vi "SeaCOM-7203.vi"() -> ()   [LabVIEW 2020]
uses:
  <vilib>/Utility/miscctls.llb/LVPointTypeDef.ctl
  LabVIEW 2020 Toolkits/toolkits_lv2020_32bit/Synchronization.llb/SynchRefs_SetGet.ctl
  LabVIEW 2020 Toolkits/VI Server Toolkit/VI Server Libraries/VI Server_GetControl.llb/VI Server_STR_Get.vi
  LabVIEW 2020 Toolkits/VI Server Toolkit/VI Server Libraries/VI Server_Set Controls.llb/Set STR Control.vi
  LabVIEW 2020 Toolkits/VI Server Toolkit/VI Server Libraries/VI Server_GetControl.llb/VI Server_1D_Array_DBL_Get.vi
  LabVIEW 2020 Toolkits/VI Server Toolkit/VI Server Libraries/VI Server_GetControl.llb/VI Server_I32_Get.vi
  LabVIEW 2020 Toolkits/VI Server Toolkit/VI Server Libraries/VI Server_SetControl.llb/VI Server_DBL_Set.vi
  LabVIEW 2020 Toolkits/VI Server Toolkit/VI Server Libraries/VI Server_SetControl.llb/VI Server_U8_Set.vi
  LabVIEW 2020 Toolkits/VI Server Toolkit/VI Server Libraries/VI Server_SetControlValue_ArrayInputs.llb/VI Server_Set U8s From ArrayInputs.vi
  LabVIEW 2020 Toolkits/VI Server Toolkit/VI Server Libraries/VI Server_SetControl.llb/VI Server_1D_STR_Set.vi
  LabVIEW 2020 Toolkits/VI Server Toolkit/VI Server Libraries/VI Server_GetControl.llb/VI Server_1D_Array_STR_Get.vi
  LabVIEW 2020 Toolkits/VI Server Toolkit/VI Server Toolkit LV2013.lvlib
panel:
  in  "Manual.Open":bool caption="IDD.Open"
  in  "IDD.Open":bool
  in  "Help":bool
  in  "FP.Hide":bool caption="FrontPanel.Hide"
  out "System.Message":string caption="System Message"
  in  "EXIT":bool
  in  "Tab.Main":T1(tab)
  out "Ch2.ReceivedDataArray.IndexedValue":dbl caption="Value" format="%0.0f"
  in  "Ch2.ReceivedDataArray.Index":i32 caption="Index" max=6
  in  "Ch2.ReceivedDataArray.Precision":u8 caption="Precision" max=6
  out "Ch2.ReceivedDataArray":dbl[](array[numeric]) caption="Received Data Array"
  out "Ch2.Responce.String":string
  out "Ch2.Responce.Payload.Num4":dbl caption="Payload Numeric 4"
  out "Ch2.Responce.Payload.Num3":dbl caption="Payload Numeric 3"
  out "Ch2.Responce.Payload.Num2":dbl caption="Payload Numeric 2"
  out "Ch2.Responce.Payload.Num1":dbl caption="Payload Numeric 1"
  out "Ch1.ReceivedDataArray.IndexedValue":dbl caption="Value" format="%0.0f"
  in  "Ch1.ReceivedDataArray.Index":i32 caption="Index" max=6
  in  "Ch1.ReceivedDataArray.Precision":u8 caption="Precision" max=6
  out "Ch1.ReceivedDataArray":dbl[](array[numeric]) caption="Received Data Array"
  out "Ch1.Responce.String":string
  out "Ch2.Responce.Message.Checksum":string caption="Checksum"
  out "Ch2.Responce.Message.Load":string caption="PayloadLoad"
  out "Ch2.Responce.Message.Length":string caption="Length"
  out "Ch2.Responce.Message.ID":string caption="Message ID"
  out "Ch2.Responce.Message.Payload":u8[](array[numeric]) caption="Message Payload" format="%02x"
  out "Ch1.Responce.Payload.Num4":dbl caption="Payload Numeric 4"
  out "Ch1.Responce.Payload.Num3":dbl caption="Payload Numeric 3"
  out "Ch1.Responce.Payload.Num2":dbl caption="Payload Numeric 2"
  out "Ch1.Responce.Payload.Num1":dbl caption="Payload Numeric 1"
  out "Ch1.Responce.Message.Checksum":string caption="Checksum"
  out "Ch1.Responce.Message.Load":string caption="PayloadLoad"
  out "Ch1.Responce.Message.Length":string caption="Length"
  out "Ch1.Responce.Message.ID":string caption="Message ID"
  out "Ch1.Responce.Message.Payload":u8[](array[numeric]) caption="Message Payload" format="%02x"
  out "StringMode.Received Data":string
  in  "Argument.Update":bool
  in  "Argument.Precision":u8 caption="Precision" max=6
  in  "Argument.Value":dbl caption="Value"
  in  "Argument.Number":i32=1 caption="Number" min=1 max=100
  in  "Message.PrototypeString":string caption="Message Prototype String"
  in  "Protocol.MessageType":u16(ring) caption="Message Type" items=["Binary", "String"]
  out "Responce.Payload.Num4":dbl caption="Payload Numeric 4"
  out "Responce.Payload.Num3":dbl caption="Payload Numeric 3"
  out "Responce.Payload.Num2":dbl caption="Payload Numeric 2"
  out "Responce.Payload.Num1":dbl caption="Payload Numeric 1"
  out "Responce.Message.Checksum":string caption="Checksum"
  out "Responce.Message.Load":string caption="PayloadLoad"
  out "Responce.Message.Length":string caption="Length"
  out "Responce.Message.ID":string caption="Message ID"
  out "Responce.Message.Payload":u8[](array[numeric]) caption="Message Payload" format="%02x"
  in  "Protocol.New":string caption="New Protocol"
  in  "Message.ItemName.Delete":bool
  in  "Protocol.ADD":bool
  in  "Protocol":u16(ring) items=["Motion Controller"]
  in  "Protocol.Delete":bool
  in  "Message.Checksum.Skip":bool
  in  "Message.Checksum":u8 caption="Checksum" format="%02x"
  in  "Message.Payload.Length":u8 caption="Payload Length" format="%02x"
  in  "Message.ID":u8 caption="ID" format="%02x"
  in  "Message.ItemName":string caption="Item Name"
  in  "Message.String.Send":bool
  in  "Message.String.Regenerate":bool
  in  "Configuration.Message.Reload":bool
  in  "Configuration.Message.SAVE":bool
  in  "Message.String":string caption="Message String"
  in  "Message.ItemName.ADD":bool caption="Message.ItemName.Update"
  in  "Message":u16(ring) caption="Messages" items=["Move Absolute Position", "Move Relative Position"]
  in  "Message.Payload":u8[](array[numeric]) caption="Message Payload" format="%02x"
  in  "Channel":u16(ring) items=["Ch1", "Ch2"]
  in  "Message.String.Send.DUP":bool caption="Message.String.Send"
  in  "Ch1.Data.Autostroll":bool
  in  "Ch1.DataReceived.Clear":bool
  in  "Ch1.DataSent.Clear":bool
  out "Ch1.DataSent":string[](array[string]) caption="Data Sent"
  out "Ch1.DataReceived":string[](array[string]) caption="Data Received"
  in  "Message.String.Send.DUP1":bool caption="Message.String.Send"
  out "Ch2.DataSent":string[](array[string]) caption="Data Sent"
  out "Ch2.DataReceived":string[](array[string]) caption="Data Received"
  in  "Ch2.DataSent.Clear":bool
  in  "Ch2.Data.Autostroll":bool
  in  "Ch2.DataReceived.Clear":bool
  in  "Conversion.U32.Byte3":u8 caption="U8: Byte 3"
  in  "Conversion.U32.Byte2":u8 caption="U8: Byte 2"
  in  "Conversion.U2.Byte1":u8 caption="U8: Byte 1"
  in  "Conversion.U32.Byte0":u8 caption="U8: Byte 0"
  in  "Conversion.U32":u16 caption="U32"
  in  "Conversion.U8.LowerByte":u8 caption="U8: Lower Byte" format="%02x"
  in  "Conversion.U8.UpperByte":u8 caption="U8: Upper Byte" format="%02x"
  in  "Conversion.U16":u16 caption="U16"
  in  "Ch2.Stop.Bits":u16(ring)=1 caption="Stop Bits" items=["1.0"=10, "1.5"=15, "2.0"=20]
  in  "Ch2.Baud.Rate":u32=115200 caption="Baud Rate"
  in  "Ch2.Data.Bits":u16=8 caption="Data Bits" min=5 max=8 step=1
  in  "Ch2.Flow.Control":u16(ring) caption="Flow Control" items=["None", "XON/XOFF", "RTS/CTS", "XON/XOFF & RTS/CTS", "DTR/DSR", "XON/XOFF & DTR/DSR"]
  in  "Ch2.Parity":u16(ring) caption="Parity" items=["None", "Odd", "Even", "Mark", "Space"]
  in  "Ch2.VISA.Resource.Name":refnum<visa-resource-name>="COM4" caption="VISA Resource Name"
  in  "Ch1.Baud.Rate":u32=115200 caption="Baud Rate"
  in  "Ch1.Data.Bits":u16=8 caption="Data Bits" min=5 max=8 step=1
  in  "Ch1.Stop.Bits":u16(ring)=1 caption="Stop Bits" items=["1.0"=10, "1.5"=15, "2.0"=20]
  in  "Ch1.Flow.Control":u16(ring) caption="Flow Control" items=["None", "XON/XOFF", "RTS/CTS", "XON/XOFF & RTS/CTS", "DTR/DSR", "XON/XOFF & DTR/DSR"]
  in  "Ch1.Parity":u16(ring) caption="Parity" items=["None", "Odd", "Even", "Mark", "Space"]
  in  "Ch1.VISA.Resource.Name":refnum<visa-resource-name>="COM3" caption="VISA Resource Name"
  in  "Setup.AdobeAcrobat.Path":path=path "C:/Program Files (x86)/Adobe/Acrobat Reader DC/Reader/AcroRd32.exe" caption="Acrobat Reader Path"
  in  "VI.WindowsTitle":string caption="Windows Title"
  in  "UDP.Test.String2.Send":bool
  in  "UDP.Test.String2":string caption="UDP: Test String 2"
  in  "UDP.Port.BC":u16=58433 caption="UDP: Port.BC"
  in  "UDP.Port.RT":u16=58432 caption="UDP: Port.RT"
  in  "UDP.LocalPort.Write":u16=58434 caption="UDP: Local Port.Write"
  in  "UDP.IP.Address":string="234.5.6.7" caption="UDP: IP Address"
  in  "UDP.Test.String1.Send":bool
  in  "UDP.Test.String1":string caption="UDP: Test String 1"
  in  "UDP.Responce.String.Monitor":bool
  out "UDP.ExecEng.Message.String":string caption="UDP: Execution Engine Message String"
  out "error out":errorcluster
  in  "error in":errorcluster
  # "Channel 1 Received Data"
  # "Channel 2 Received Data"
  # "Received Data"
  # "Channel 2"
  # "Channel 1"
  # "Multicast IP addresses must be in the 224.0.0.0 to 239.255.255.255 range."
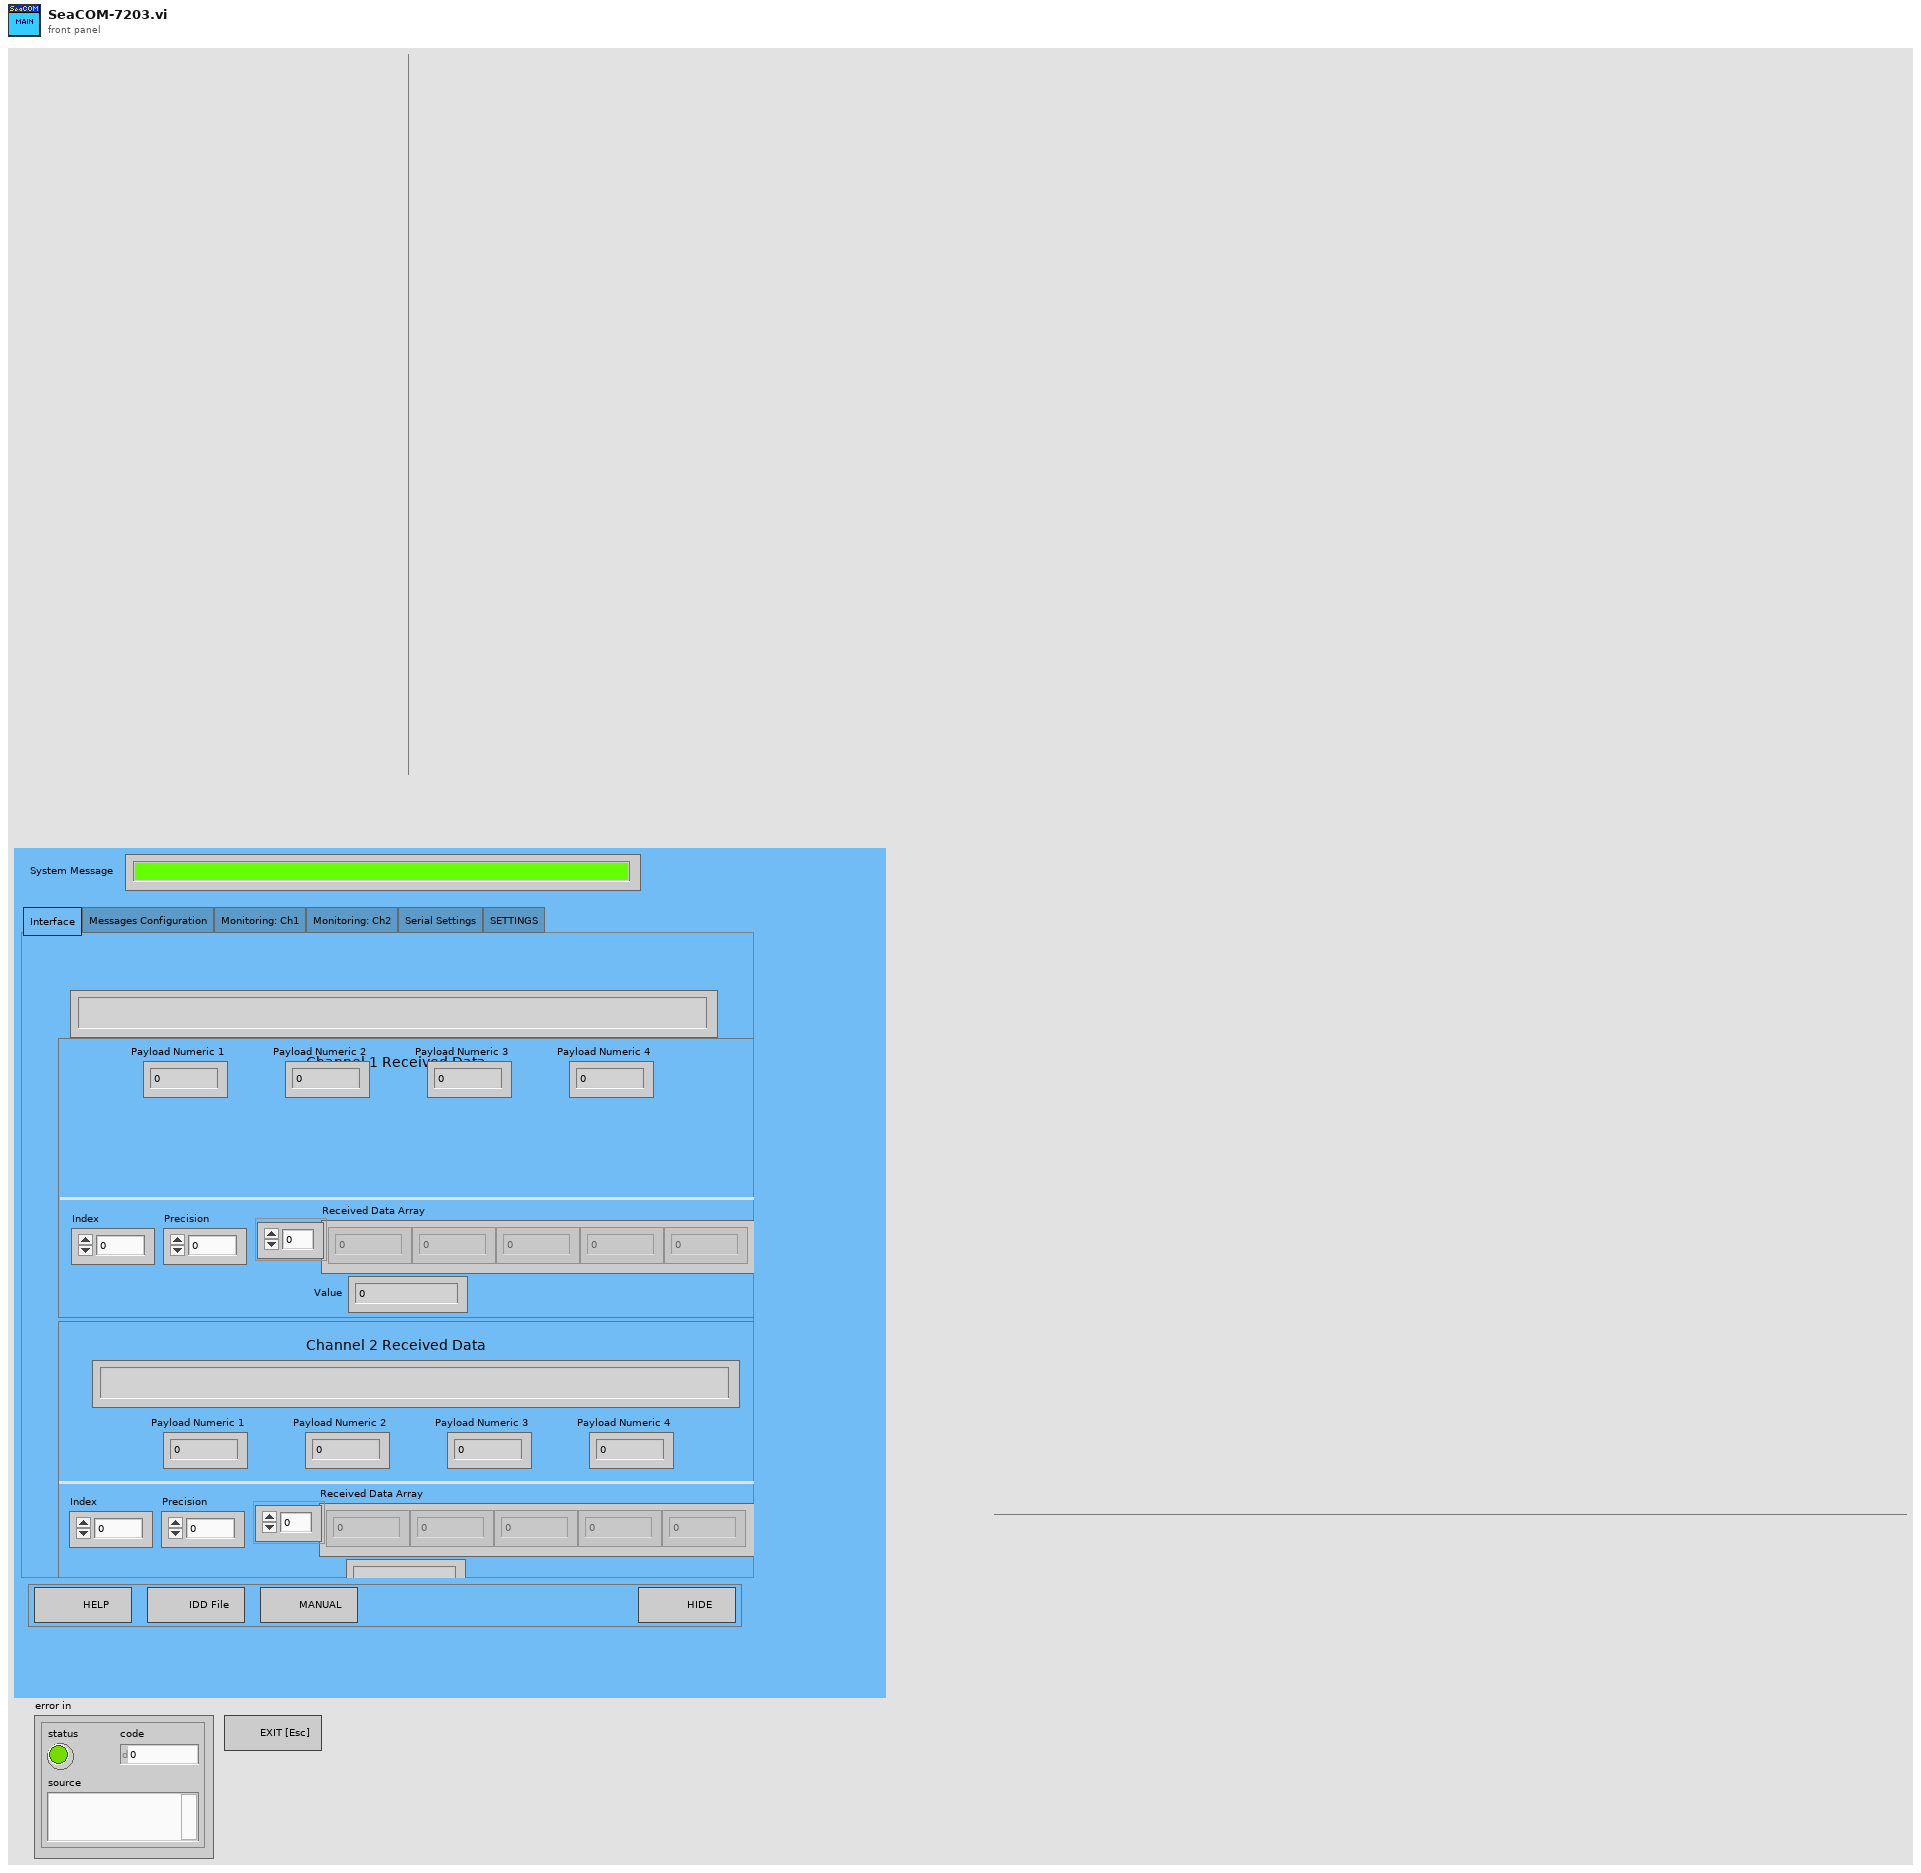
[diagram p1: front panel]
types:
  T1 = enum32{"Interface", "Messages Configuration", "Monitoring: Ch1", "Monitoring: Ch2", "Serial Settings", "SETTINGS"}
  T2 = typedef "LVPointTypeDef.ctl" = cluster{"Horizontal":i16, "Vertical":i16}
  T3 = typedef "VI Server_RefsCluster.ctl" = cluster{"Labels":string[], "Refs":refnum<vi>[], "VI Ref":refnum<vi>}
  T4 = typedef "SynchRefs_SetGet.ctl" = enum16{"Set", "Get"}
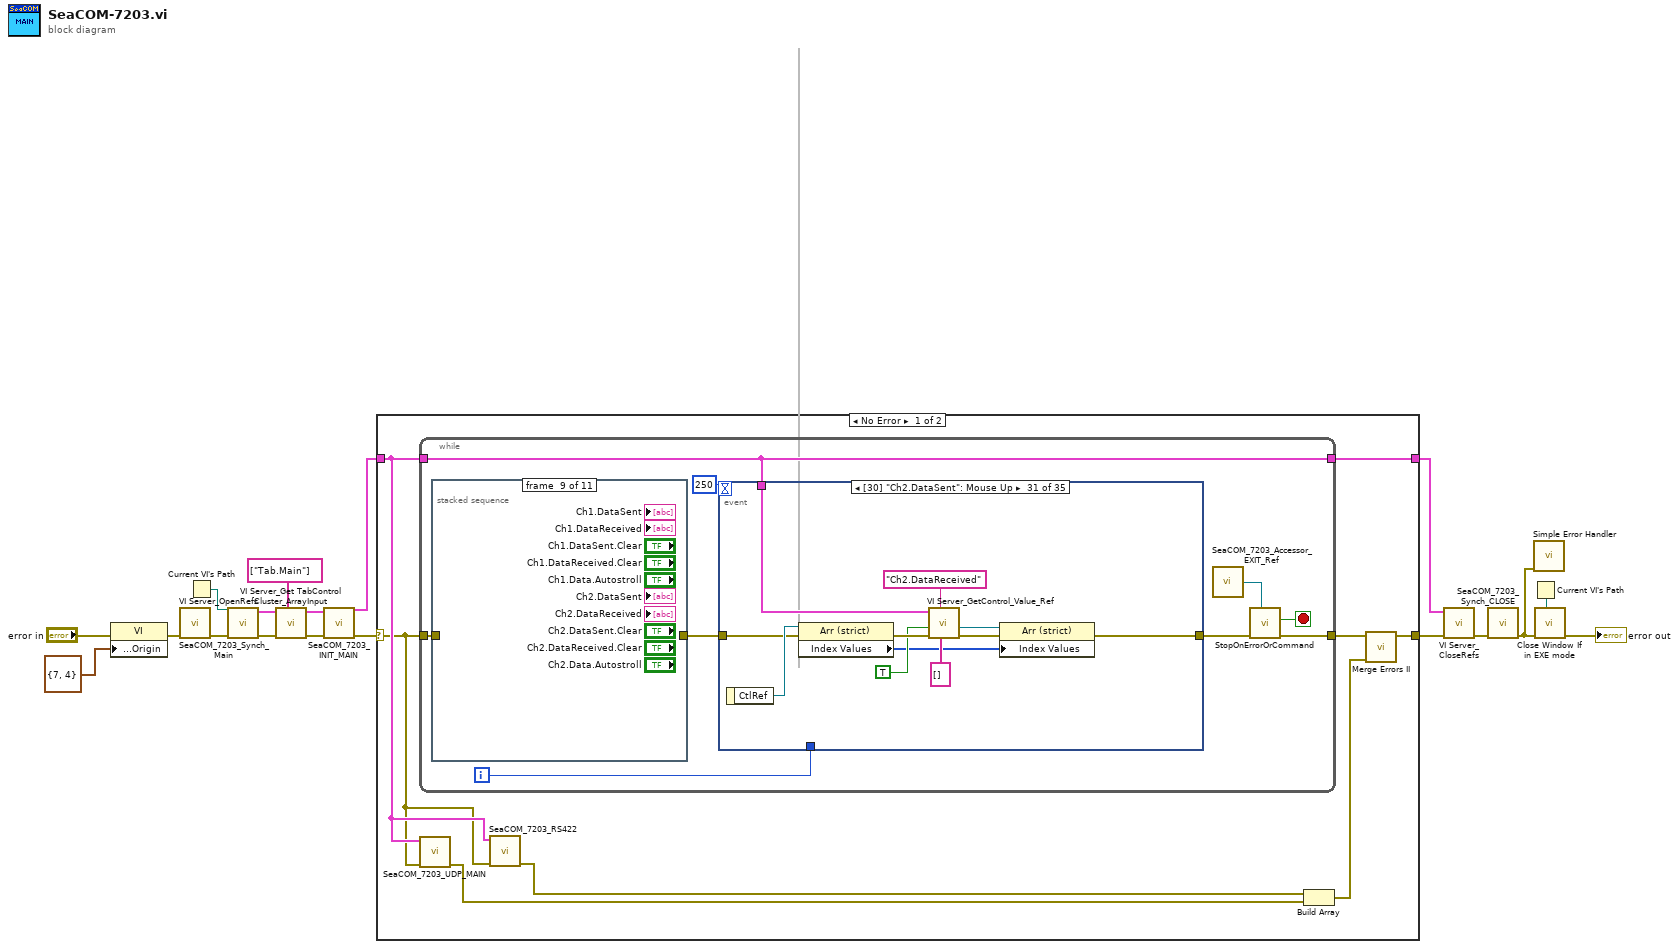
[diagram p0: block diagram]
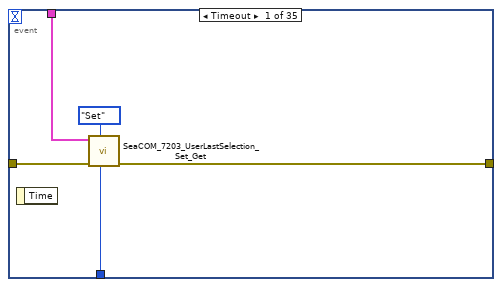
[diagram p2: hidden frame]
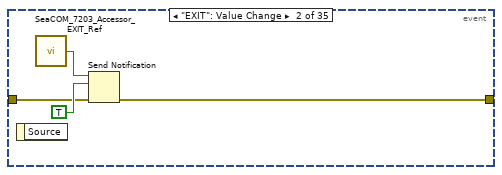
[diagram p3: hidden frame]
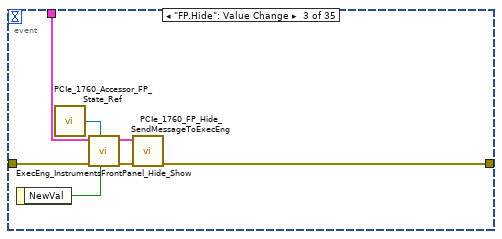
[diagram p4: hidden frame]
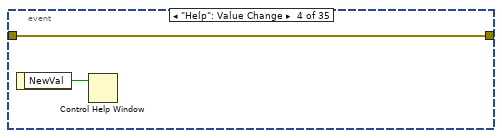
[diagram p5: hidden frame]
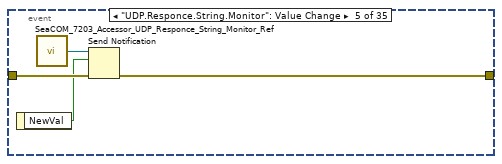
[diagram p6: hidden frame]
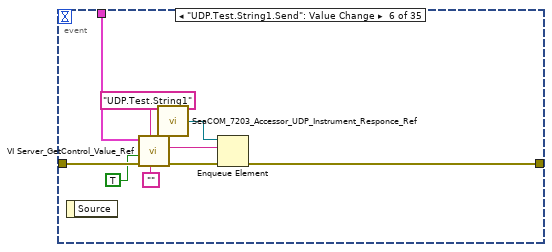
[diagram p7: hidden frame]
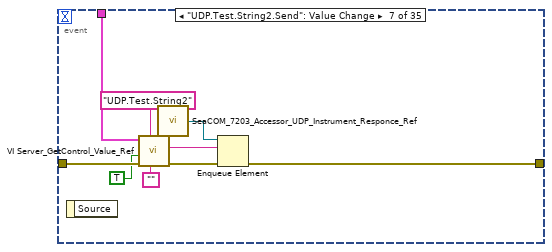
[diagram p8: hidden frame]
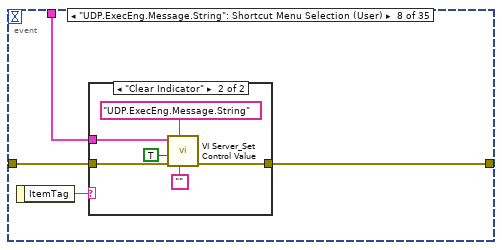
[diagram p9: hidden frame]
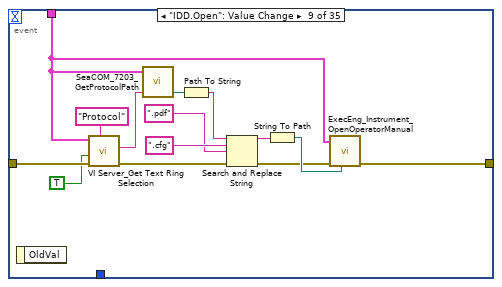
[diagram p11: hidden frame]
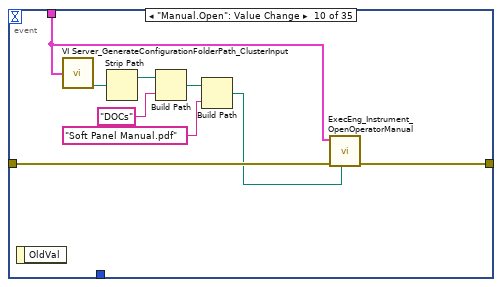
[diagram p12: hidden frame]
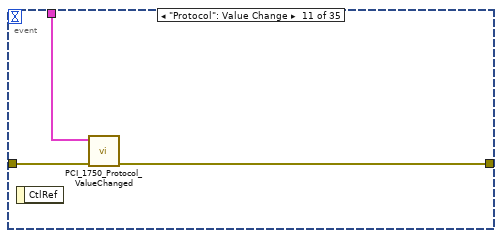
[diagram p13: hidden frame]
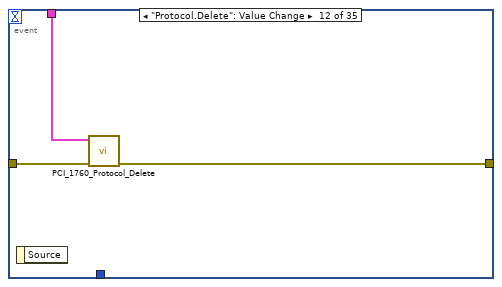
[diagram p14: hidden frame]
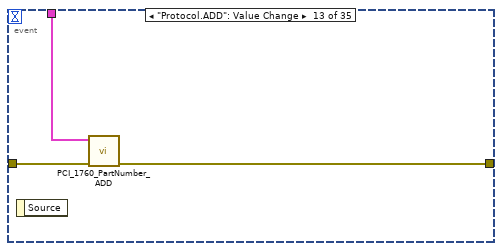
[diagram p15: hidden frame]
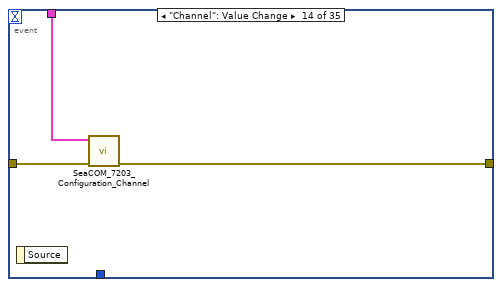
[diagram p16: hidden frame]
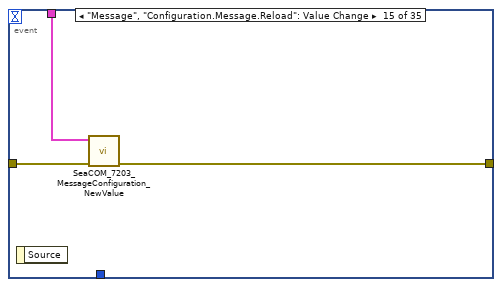
[diagram p17: hidden frame]
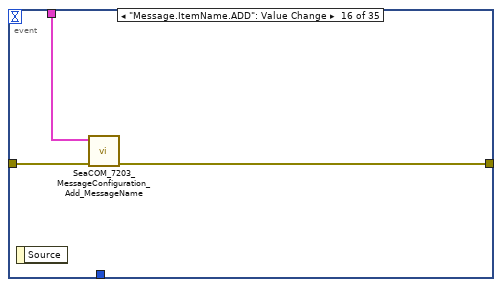
[diagram p18: hidden frame]
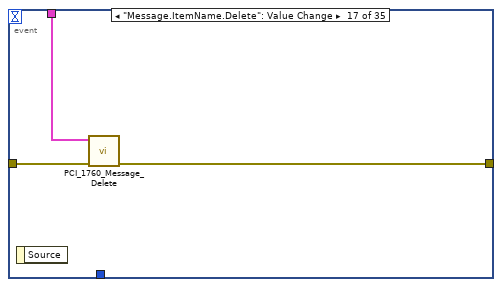
[diagram p19: hidden frame]
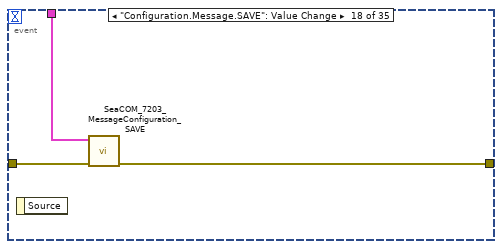
[diagram p20: hidden frame]
diagram:
  n1 = property class="VI"(error in="error in", "Front Panel Window:Origin"=T2 {"Horizontal"=7, "Vertical"=4}) -> (error out=w12:errorcluster)  [unwired: 1 in, 1 out]
  n2 = call "SeaCOM_7203_Synch_Main.vi"("error in"=w12) -> ("error out"=w13:errorcluster)  [unwired: 10 in]
  n3 = Current VI's Path() -> (path=w17:path)
  n4 = call "VI Server_OpenRefs.vi"("error in"=w13, "VI Path"=w17) -> ("error out"=w14:errorcluster, "VI Server.RefsCluster"=w15:T3)  [unwired: 8 in]
  n5 = call "VI Server_Get TabControl Cluster_ArrayInput.vi"("TabControl Labels[]"=string[] ["Tab.Main"], "error in"=w14, "VI Server Cluster"=w15) -> ("error out"=w11:errorcluster, "VI Server Cluster.OUT"=w10:T3)  [unwired: 7 in]
  n6 = call "SeaCOM_7203_INIT_MAIN.vi"("error in (no error)"=w11, "VI Server Cluster"=w10) -> ("error out"=w9:errorcluster, "VI Server Cluster DUP"=w8:T3)  [unwired: 8 in]
  n7 = case shown="No Error" w9 {
    selector: w9 -> [w20 w303]
    tunnel: [w23 w303] -> w2
    tunnel: w8 -> [w21 w302]
    tunnel: [w26 w302] -> w3
    frame No Error {
      n8 = while {
        tunnel: w20 -> [w35]
        tunnel: [w29] -> w24
        tunnel: w21 -> [w31]
        tunnel: [w31] -> w26
        i -> [w32]
        stop <- w28 stop-if-true
        n9 = stacked-sequence {
          tunnel: w35 -> [w301 _ _ _ _ _ _ _ _ _ _]
          tunnel: [w301 _ _ _ _ _ _ _ _ _ _] -> w34
          frame #0 {
          }
          frame #1 {
          }
          frame #2 {
          }
          frame #3 {
          }
          frame #4 {
          }
          frame #5 {
          }
          frame #6 {
          }
          frame #7 {
          }
          frame #8 {
          }
          frame #9 {
          }
          frame #10 {
          }
        }
        n10 = event shown="[30] \"Ch2.DataSent\": Mouse Up" {
          selector: _ -> [_ _ _ _ _ _ _ _ _ _ _ _ _ _ _ _ _ _ _ _ _ _ _ _ _ _ _ _ _ _ _ _ _ _ _]
          dyn-events: _ -> [_ _ _ _ _ _ _ _ _ _ _ _ _ _ _ _ _ _ _ _ _ _ _ _ _ _ _ _ _ _ _ _ _ _ _]
          timeout: 250 -> [_ _ _ _ _ _ _ _ _ _ _ _ _ _ _ _ _ _ _ _ _ _ _ _ _ _ _ _ _ _ _ _ _ _ _]
          tunnel: w34 -> [w39 w41 w50 w53 w57 w66 w75 w79 w99 w108 w110 w115 w118 w121 w124 w127 w130 w133 w136 w139 w155 w171 w173 w184 w191 w207 w216 w225 w234 w244 w255 w266 w277 w288 w299]
          tunnel: w32 -> [w38 _ _ _ _ _ _ _ _ _ _ _ _ _ _ _ _ _ _ _ _ _ _ _ _ _ _ _ _ _ _ _ _ _ _]
          tunnel: [w36 w43 w51 w53 w55 w64 w73 w77 w100 w109 w111 w114 w116 w119 w122 w125 w128 w132 w135 w138 w140 w156 w174 w179 w189 w201 w210 w219 w226 w236 w247 w258 w269 w280 w291] -> w30
          tunnel: w31 -> [w37 _ w47 _ _ w63 w72 w76 w98 w107 w112 w113 w117 w120 w123 w126 w129 w131 w134 w137 w154 w170 w172 w183 w190 w206 w215 w224 w233 w241 w252 w263 w274 w285 w296]
          event Timeout {
            n11 = event-data() -> ()  [unwired: 1 in, 1 out]
            n12 = call "SeaCOM_7203_UserLastSelection_Set_Get.vi"("LoopCounter"=w38, "SynchRefs.Set/Get"=SynchRefs_SetGet."Set", "error in"=w39, "VI Server.RefsCluster"=w37) -> ("error out"=w36:errorcluster)  [unwired: 6 in, 1 out]
          }
          event "EXIT": Value Change {
            n13 = event-data() -> ()  [unwired: 1 in, 1 out]
            n14 = call "SeaCOM_7203_Accessor_EXIT_Ref.vi"() -> ("EXIT"=w44:refnum<notifier>)  [unwired: 6 in]
            n15 = Send Notification(notification=TRUE, notifier=w44, error in (no error)=w41) -> (error out=w43:errorcluster)  [unwired: 1 out]
          }
          event "FP.Hide": Value Change {
            n16 = event-data() -> ("NewVal"=w48:bool)  [unwired: 1 in]
            n17 = call "PCIe_1760_Accessor_FP_State_Ref.vi"() -> ("FP.State"=w45:refnum<notifier>)  [unwired: 6 in]
            n18 = call "ExecEng_InstrumentsFrontPanel_Hide_Show.vi"("FP.Hide/Show"=w48, "FP.State"=w45, "error in (no error)"=w50, "VI Server Cluster"=w47) -> ("error out"=w49:errorcluster, "VI Server Cluster DUP"=w46:T3)  [unwired: 6 in]
            n19 = call "PCIe_1760_FP_Hide_SendMessageToExecEng.vi"("error in (no error)"=w49, "VI Server Cluster"=w46) -> ("error out"=w51:errorcluster)  [unwired: 9 in]
          }
          event "Help": Value Change {
            n20 = event-data() -> ("NewVal"=w52:bool)  [unwired: 1 in]
            n21 = Control Help Window(1:w52) -> ()  [unwired: 1 in]
          }
          event "UDP.Responce.String.Monitor": Value Change {
            n22 = event-data() -> ("NewVal"=w54:bool)  [unwired: 1 in]
            n23 = call "SeaCOM_7203_Accessor_UDP_Responce_String_Monitor_Ref.vi"() -> ("UDP.ExecEng.Command.String.Monitor"=w56:refnum<notifier>)  [unwired: 6 in]
            n24 = Send Notification(notification=w54, notifier=w56, error in (no error)=w57) -> (error out=w55:errorcluster)  [unwired: 1 out]
          }
          event "UDP.Test.String1.Send": Value Change {
            n25 = event-data() -> ()  [unwired: 1 in, 1 out]
            n26 = call-poly "VI Server_GetControl_Value_Ref.vi"("DataType"="", "Control.Label"="UDP.Test.String1", "error in"=w66, "SingleInstance"=TRUE, "VI Server.RefsCluster"=w63) -> ("error out"=w65:errorcluster, "Value"=w58:string)  [unwired: 3 in, 2 out]
            n27 = call "SeaCOM_7203_Accessor_UDP_Instrument_Responce_Ref.vi"() -> ("UDP.Instrument.Responce.Q"=w59:refnum<queue>)  [unwired: 6 in]
            n28 = Enqueue Element(queue=w59, element=w58, error in (no error)=w65) -> (error out=w64:errorcluster)  [unwired: 1 in, 2 out]
          }
          event "UDP.Test.String2.Send": Value Change {
            n29 = event-data() -> ()  [unwired: 1 in, 1 out]
            n30 = call-poly "VI Server_GetControl_Value_Ref.vi"("DataType"="", "Control.Label"="UDP.Test.String2", "error in"=w75, "SingleInstance"=TRUE, "VI Server.RefsCluster"=w72) -> ("error out"=w74:errorcluster, "Value"=w67:string)  [unwired: 3 in, 2 out]
            n31 = call "SeaCOM_7203_Accessor_UDP_Instrument_Responce_Ref.vi"() -> ("UDP.Instrument.Responce.Q"=w68:refnum<queue>)  [unwired: 6 in]
            n32 = Enqueue Element(queue=w68, element=w67, error in (no error)=w74) -> (error out=w73:errorcluster)  [unwired: 1 in, 2 out]
          }
          event "UDP.ExecEng.Message.String": Shortcut Menu Selection (User) {
            n33 = event-data() -> ("ItemTag"=w78:string)  [unwired: 1 in]
            n34 = case shown="\"Clear Indicator\"" w78 {
              tunnel: w79 -> [w80 w86]
              tunnel: [w80 w85] -> w77
              tunnel: w76 -> [_ w84]
              frame "", Default {
              }
              frame "Clear Indicator" {
                n35 = call-poly "VI Server_Set Control Value.vi"("New Value"="", "Label"="UDP.ExecEng.Message.String" ("Control.Label"), "error in"=w86, "Single Instance (T)"=TRUE ("SingleInstance"), "VI Server Cluster"=w84) -> ("error out"=w85:errorcluster)  [unwired: 4 in, 2 out]
              }
            }
          }
          event "IDD.Open": Value Change {
            n36 = event-data() -> ()  [unwired: 1 in, 1 out]
            n37 = call "VI Server_Get Text Ring Selection.vi"("Label"="Protocol", "error in"=w99, "Single Instance (T)"=TRUE, "VI Server Cluster"=w98) -> ("error out"=w88:errorcluster, "Selection"=w95:string)  [unwired: 2 in, 4 out]
            n38 = call "SeaCOM_7203_GetProtocolPath.vi"("VI Server Cluster"=w98, "Protocol.Name"=w95) -> ("Protocol.Path"=w94:path)  [unwired: 3 in, 2 out]
            n39 = Path To String(path=w94) -> (string=w93:string)
            n40 = Search and Replace String(input string=w93, search string=".cfg", replace string=".pdf" ("replace string (\"\")"), error in=w88) -> (result string=w90:string, error out=w87:errorcluster)  [unwired: 4 in, 2 out]
            n41 = String To Path(string=w90) -> (path=w89:path)
            n42 = call "ExecEng_Instrument_OpenOperatorManual.vi"("Operations Manual Path"=w89, "error in"=w87, "VI Server.RefsCluster"=w98) -> ("error out"=w100:errorcluster)  [unwired: 8 in]
          }
          event "Manual.Open": Value Change {
            n43 = event-data() -> ()  [unwired: 1 in, 1 out]
            n44 = call "VI Server_GenerateConfigurationFolderPath_ClusterInput.vi"("VI Server Cluster"=w107) -> ("Configuration Folder Path"=w106:path)  [unwired: 11 in, 3 out]
            n45 = Strip Path(path=w106) -> (stripped path=w105:path)  [unwired: 1 out]
            n46 = Build Path(base path=w105, name or relative path="DOCs") -> (appended path=w103:path)
            n47 = Build Path(base path=w103, name or relative path="Soft Panel Manual.pdf") -> (appended path=w101:path)
            n48 = call "ExecEng_Instrument_OpenOperatorManual.vi"("Operations Manual Path"=w101, "error in"=w108, "VI Server.RefsCluster"=w107) -> ("error out"=w109:errorcluster)  [unwired: 8 in]
          }
          event "Protocol": Value Change {
            n49 = event-data() -> ()  [unwired: 1 in, 1 out]
            n50 = call "PCI_1750_Protocol_ValueChanged.vi"("error in (no error)"=w110, "VI Server Cluster"=w112) -> ("error out"=w111:errorcluster)  [unwired: 8 in, 1 out]
          }
          event "Protocol.Delete": Value Change {
            n51 = event-data() -> ()  [unwired: 1 in, 1 out]
            n52 = call "PCI_1760_Protocol_Delete.vi"("error in (no error)"=w115, "VI Server Cluster"=w113) -> ("error out"=w114:errorcluster)  [unwired: 9 in]
          }
          event "Protocol.ADD": Value Change {
            n53 = event-data() -> ()  [unwired: 1 in, 1 out]
            n54 = call "PCI_1760_PartNumber_ADD.vi"("error in (no error)"=w118, "VI Server Cluster"=w117) -> ("error out"=w116:errorcluster)  [unwired: 9 in]
          }
          event "Channel": Value Change {
            n55 = event-data() -> ()  [unwired: 1 in, 1 out]
            n56 = call "SeaCOM_7203_Configuration_Channel.vi"("error in (no error)"=w121, "VI Server Cluster"=w120) -> ("error out"=w119:errorcluster)  [unwired: 9 in]
          }
          event "Message", "Configuration.Message.Reload": Value Change {
            n57 = event-data() -> ()  [unwired: 1 in, 1 out]
            n58 = call "SeaCOM_7203_MessageConfiguration_NewValue.vi"("error in (no error)"=w124, "VI Server Cluster"=w123) -> ("error out"=w122:errorcluster)  [unwired: 9 in]
          }
          event "Message.ItemName.ADD": Value Change {
            n59 = event-data() -> ()  [unwired: 1 in, 1 out]
            n60 = call "SeaCOM_7203_MessageConfiguration_Add_MessageName.vi"("error in (no error)"=w127, "VI Server Cluster"=w126) -> ("error out"=w125:errorcluster)  [unwired: 9 in]
          }
          event "Message.ItemName.Delete": Value Change {
            n61 = event-data() -> ()  [unwired: 1 in, 1 out]
            n62 = call "PCI_1760_Message_Delete.vi"("error in (no error)"=w130, "VI Server Cluster"=w129) -> ("error out"=w128:errorcluster)  [unwired: 9 in]
          }
          event "Configuration.Message.SAVE": Value Change {
            n63 = event-data() -> ()  [unwired: 1 in, 1 out]
            n64 = call "SeaCOM_7203_MessageConfiguration_SAVE.vi"("error in (no error)"=w133, "VI Server Cluster"=w131) -> ("error out"=w132:errorcluster)  [unwired: 9 in]
          }
          event "Message.ID", "Message.Payload", "Message.String.Regenerate": Value Change {
            n65 = event-data() -> ()  [unwired: 1 in, 1 out]
            n66 = call "SeaCOM_7203_FormatMessageString.vi"("error in (no error)"=w136, "VI Server Cluster"=w134) -> ("error out"=w135:errorcluster)  [unwired: 9 in]
          }
          event "Argument.Update": Value Change {
            n67 = event-data() -> ()  [unwired: 1 in, 2 out]
            n68 = call "SeaCOM_7203_StringProtocol_Update.vi"("error in (no error)"=w139, "VI Server Cluster"=w137) -> ("error out"=w138:errorcluster)  [unwired: 9 in]
          }
          event "Ch2.ReceivedDataArray.Index": Value Change {
            w142 = TRUE ("SingleInstance")
            n69 = event-data() -> ()  [unwired: 1 in, 2 out]
            n70 = call-poly "VI Server_GetControl_Value_Ref.vi"("DataType"=dbl[] [], "Control.Label"="Ch2.ReceivedDataArray", "error in"=w155, "SingleInstance"=w142, "VI Server.RefsCluster"=w154) -> ("error out"=w151:errorcluster, "Value"=w148:dbl[], "VI Server.RefsCluster.DUP"=w150:T3)  [unwired: 3 in, 1 out]
            n71 = call-poly "VI Server_GetControl_Value_Ref.vi"("DataType"=0, "Control.Label"="Ch2.ReceivedDataArray.Index", "error in"=w151, "SingleInstance"=w142, "VI Server.RefsCluster"=w150) -> ("error out"=w143:errorcluster, "Value"=w146:i32, "VI Server.RefsCluster.DUP"=w145:T3)  [unwired: 3 in, 1 out]
            n72 = Index Array(array=w148, index=w146) -> (element=w144:dbl)
            n73 = call-poly "VI Server_SetControl.vi"("Data"=w144, "Control.Label"="Ch2.ReceivedDataArray.IndexedValue", "error in"=w143, "SingleInstance"=w142, "VI Server.RefsCluster"=w145) -> ("error out"=w140:errorcluster)  [unwired: 4 in, 2 out]
          }
          event "Ch1.ReceivedDataArray.Index": Value Change {
            w158 = TRUE ("SingleInstance")
            n74 = event-data() -> ()  [unwired: 1 in, 2 out]
            n75 = call-poly "VI Server_GetControl_Value_Ref.vi"("DataType"=dbl[] [], "Control.Label"="Ch1.ReceivedDataArray", "error in"=w171, "SingleInstance"=w158, "VI Server.RefsCluster"=w170) -> ("error out"=w167:errorcluster, "Value"=w164:dbl[], "VI Server.RefsCluster.DUP"=w166:T3)  [unwired: 3 in, 1 out]
            n76 = call-poly "VI Server_GetControl_Value_Ref.vi"("DataType"=0, "Control.Label"="Ch1.ReceivedDataArray.Index", "error in"=w167, "SingleInstance"=w158, "VI Server.RefsCluster"=w166) -> ("error out"=w159:errorcluster, "Value"=w162:i32, "VI Server.RefsCluster.DUP"=w161:T3)  [unwired: 3 in, 1 out]
            n77 = Index Array(array=w164, index=w162) -> (element=w160:dbl)
            n78 = call-poly "VI Server_SetControl.vi"("Data"=w160, "Control.Label"="Ch1.ReceivedDataArray.IndexedValue", "error in"=w159, "SingleInstance"=w158, "VI Server.RefsCluster"=w161) -> ("error out"=w156:errorcluster)  [unwired: 4 in, 2 out]
          }
          event "Message.String.Send", "Message.String.Send.DUP", "Message.String.Send.DUP1": Value Change {
            n79 = event-data() -> ()  [unwired: 1 in, 1 out]
            n80 = call "SeaCOM_7203_Configuration_ChannelMessage_Write.vi"("error in (no error)"=w173, "VI Server Cluster"=w172) -> ("error out"=w174:errorcluster)  [unwired: 9 in]
          }
          event "Conversion.U16": Value Change {
            w178 = TRUE ("SingleInstance")
            n81 = event-data() -> ("NewVal"=w185:u16)  [unwired: 1 in]
            n82 = Split Number(x=w185) -> (hi(x)=w181:u8, lo(x)=w175:u8)
            n83 = call-poly "VI Server_SetControl.vi"("Data"=w181, "Control.Label"="Conversion.U8.UpperByte", "error in"=w184, "SingleInstance"=w178, "VI Server.RefsCluster"=w183) -> ("error out"=w180:errorcluster, "VI Server.RefsCluster.DUP"=w177:T3)  [unwired: 4 in, 1 out]
            n84 = call-poly "VI Server_SetControl.vi"("Data"=w175, "Control.Label"="Conversion.U8.LowerByte", "error in"=w180, "SingleInstance"=w178, "VI Server.RefsCluster"=w177) -> ("error out"=w179:errorcluster)  [unwired: 4 in, 2 out]
          }
          event "Conversion.U32": Value Change {
            n85 = event-data() -> ("NewVal"=w198:u16)  [unwired: 1 in]
            n86 = Split Number(x=w198) -> (hi(x)=w196:u8, lo(x)=w197:u8)
            n87 = Split Number(x=w196) -> (hi(x)=w195:u8, lo(x)=w194:u8)
            n88 = Split Number(x=w197) -> (hi(x)=w193:u8, lo(x)=w192:u8)
            n89 = Build Array(w195, w194, w193, w192) -> (w188:u8[])
            n90 = call-poly "VI Server_SetControls_ArrayInputs.vi"("[New Data]"=w188, "New Data"=u8 0, "Labels Array"=string[] ["Conversion.U32.Byte0", "Conversion.U2.Byte1", "Conversion.U32.Byte2", "Conversion.U32.Byte3"], "error in (no error)"=w191, "VI Server Cluster"=w190) -> ("error out"=w189:errorcluster)  [unwired: 5 in, 1 out]
          }
          event "Ch1.DataSent.Clear": Value Change {
            n91 = event-data() -> ()  [unwired: 1 in, 1 out]
            n92 = call-poly "VI Server_SetControl.vi"("Data"=string[] [], "Control.Label"="Ch1.DataSent" ("Label"), "error in"=w207, "SingleInstance"=TRUE, "VI Server.RefsCluster"=w206) -> ("error out"=w202:errorcluster, "Control.Ref"=w200:refnum<vi>)  [unwired: 4 in, 1 out]
            n93 = property class="Arr (strict)"(reference=w200, error in=w202, "Index Values"=u32[] [0]) -> (error out=w201:errorcluster)  [unwired: 1 out]
          }
          event "Ch2.DataSent.Clear": Value Change {
            n94 = event-data() -> ()  [unwired: 1 in, 1 out]
            n95 = call-poly "VI Server_SetControl.vi"("Data"=string[] [], "Control.Label"="Ch2.DataSent" ("Label"), "error in"=w216, "SingleInstance"=TRUE, "VI Server.RefsCluster"=w215) -> ("error out"=w211:errorcluster, "Control.Ref"=w209:refnum<vi>)  [unwired: 4 in, 1 out]
            n96 = property class="Arr (strict)"(reference=w209, error in=w211, "Index Values"=u32[] [0]) -> (error out=w210:errorcluster)  [unwired: 1 out]
          }
          event "Ch2.DataReceived.Clear": Value Change {
            n97 = event-data() -> ()  [unwired: 1 in, 1 out]
            n98 = call-poly "VI Server_SetControl.vi"("Data"=string[] [], "Control.Label"="Ch2.DataReceived" ("Label"), "error in"=w225, "SingleInstance"=TRUE, "VI Server.RefsCluster"=w224) -> ("error out"=w220:errorcluster, "Control.Ref"=w218:refnum<vi>)  [unwired: 4 in, 1 out]
            n99 = property class="Arr (strict)"(reference=w218, error in=w220, "Index Values"=u32[] [0]) -> (error out=w219:errorcluster)  [unwired: 1 out]
          }
          event "Ch1.DataReceived.Clear": Value Change {
            n100 = event-data() -> ()  [unwired: 1 in, 1 out]
            n101 = call-poly "VI Server_SetControl.vi"("Data"=string[] [], "Control.Label"="Ch1.DataReceived" ("Label"), "error in"=w234, "SingleInstance"=TRUE, "VI Server.RefsCluster"=w233) -> ("error out"=w227:errorcluster, "Control.Ref"=w228:refnum<vi>)  [unwired: 4 in, 1 out]
            n102 = property class="Arr (strict)"(reference=w228, error in=w227, "Index Values"=u32[] [0]) -> (error out=w226:errorcluster)  [unwired: 1 out]
          }
          event "Ch1.DataSent": Mouse Up {
            n103 = event-data() -> ("CtlRef"=w245:refnum<vi>)  [unwired: 1 in]
            n104 = property class="Arr (strict)"(reference=w245, error in=w244) -> (error out=w243:errorcluster, "Index Values"=w235:u32[])  [unwired: 1 out]
            n105 = call-poly "VI Server_GetControl_Value_Ref.vi"("DataType"=string[] [], "Control.Label"="Ch1.DataReceived", "error in"=w243, "SingleInstance"=TRUE, "VI Server.RefsCluster"=w241) -> ("error out"=w238:errorcluster, "Control.Ref"=w237:refnum<vi>)  [unwired: 3 in, 2 out]
            n106 = property class="Arr (strict)"(reference=w237, error in=w238, "Index Values"=w235) -> (error out=w236:errorcluster)  [unwired: 1 out]
          }
          event "Ch2.DataSent": Mouse Up {
            n107 = event-data() -> ("CtlRef"=w256:refnum<vi>)  [unwired: 1 in]
            n108 = property class="Arr (strict)"(reference=w256, error in=w255) -> (error out=w254:errorcluster, "Index Values"=w246:u32[])  [unwired: 1 out]
            n109 = call-poly "VI Server_GetControl_Value_Ref.vi"("DataType"=string[] [], "Control.Label"="Ch2.DataReceived", "error in"=w254, "SingleInstance"=TRUE, "VI Server.RefsCluster"=w252) -> ("error out"=w249:errorcluster, "Control.Ref"=w248:refnum<vi>)  [unwired: 3 in, 2 out]
            n110 = property class="Arr (strict)"(reference=w248, error in=w249, "Index Values"=w246) -> (error out=w247:errorcluster)  [unwired: 1 out]
          }
          event "Ch2.DataReceived": Mouse Up {
            n111 = event-data() -> ("CtlRef"=w267:refnum<vi>)  [unwired: 1 in]
            n112 = property class="Arr (strict)"(reference=w267, error in=w266) -> (error out=w265:errorcluster, "Index Values"=w257:u32[])  [unwired: 1 out]
            n113 = call-poly "VI Server_GetControl_Value_Ref.vi"("DataType"=string[] [], "Control.Label"="Ch2.DataSent", "error in"=w265, "SingleInstance"=TRUE, "VI Server.RefsCluster"=w263) -> ("error out"=w260:errorcluster, "Control.Ref"=w259:refnum<vi>)  [unwired: 3 in, 2 out]
            n114 = property class="Arr (strict)"(reference=w259, error in=w260, "Index Values"=w257) -> (error out=w258:errorcluster)  [unwired: 1 out]
          }
          event "Ch1.DataReceived": Mouse Up {
            n115 = event-data() -> ("CtlRef"=w278:refnum<vi>)  [unwired: 1 in]
            n116 = property class="Arr (strict)"(reference=w278, error in=w277) -> (error out=w276:errorcluster, "Index Values"=w268:u32[])  [unwired: 1 out]
            n117 = call-poly "VI Server_GetControl_Value_Ref.vi"("DataType"=string[] [], "Control.Label"="Ch1.DataSent", "error in"=w276, "SingleInstance"=TRUE, "VI Server.RefsCluster"=w274) -> ("error out"=w271:errorcluster, "Control.Ref"=w270:refnum<vi>)  [unwired: 3 in, 2 out]
            n118 = property class="Arr (strict)"(reference=w270, error in=w271, "Index Values"=w268) -> (error out=w269:errorcluster)  [unwired: 1 out]
          }
          event "Ch2.DataSent": Value Change {
            n119 = event-data() -> ("CtlRef"=w289:refnum<vi>)  [unwired: 1 in]
            n120 = property class="Arr (strict)"(reference=w289, error in=w288) -> (error out=w287:errorcluster, "Index Values"=w279:u32[])  [unwired: 1 out]
            n121 = call-poly "VI Server_GetControl_Value_Ref.vi"("DataType"=string[] [], "Control.Label"="Ch2.DataReceived", "error in"=w287, "SingleInstance"=TRUE, "VI Server.RefsCluster"=w285) -> ("error out"=w282:errorcluster, "Control.Ref"=w281:refnum<vi>)  [unwired: 3 in, 2 out]
            n122 = property class="Arr (strict)"(reference=w281, error in=w282, "Index Values"=w279) -> (error out=w280:errorcluster)  [unwired: 1 out]
          }
          event "Ch2.DataReceived": Value Change {
            n123 = event-data() -> ("CtlRef"=w300:refnum<vi>)  [unwired: 1 in]
            n124 = property class="Arr (strict)"(reference=w300, error in=w299) -> (error out=w298:errorcluster, "Index Values"=w290:u32[])  [unwired: 1 out]
            n125 = call-poly "VI Server_GetControl_Value_Ref.vi"("DataType"=string[] [], "Control.Label"="Ch2.DataSent", "error in"=w298, "SingleInstance"=TRUE, "VI Server.RefsCluster"=w296) -> ("error out"=w293:errorcluster, "Control.Ref"=w292:refnum<vi>)  [unwired: 3 in, 2 out]
            n126 = property class="Arr (strict)"(reference=w292, error in=w293, "Index Values"=w290) -> (error out=w291:errorcluster)  [unwired: 1 out]
          }
        }
        n127 = call "SeaCOM_7203_Accessor_EXIT_Ref.vi"() -> ("EXIT"=w27:refnum<notifier>)  [unwired: 6 in]
        n128 = call "StopOnErrorOrCommand.vi"("STOP"=w27, "error in (no error)"=w30) -> ("error out"=w29:errorcluster, "STOP"=w28:bool)  [unwired: 8 in]
      }
      n129 = call "SeaCOM_7203_UDP_MAIN.vi"("error in (no error)"=w20, "VI Server.RefsCluster"=w21) -> ("error out"=w25:errorcluster)  [unwired: 9 in]
      n130 = call "SeaCOM_7203_RS422.vi"("error in (no error)"=w20, "VI Server Cluster"=w21) -> ("error out"=w19:errorcluster)  [unwired: 9 in]
      n131 = Build Array(w19, w25) -> (w22:errorcluster[])
      n132 = call "Merge Errors II.vi"("error array in"=w22, "error in 1 (no error)"=w24) -> ("error out.DUP"=w23:errorcluster)  [unwired: 4 in, 1 out]
    }
    frame Error {
    }
  }
  n133 = call "VI Server_CloseRefs.vi"("error in"=w2, "VI Server.RefsCluster"=w3) -> ("error out"=w7:errorcluster)  [unwired: 9 in]
  n134 = call "SeaCOM_7203_Synch_CLOSE.vi"("error in"=w7) -> ("error out"=w1:errorcluster)  [unwired: 10 in]
  n135 = Current VI's Path() -> (path=w5:path)
  n136 = call <vilib>:"Simple Error Handler.vi"("error in (no error)"=w1) -> ()  [unwired: 4 in, 5 out]
  n137 = call "Close Window If in EXE mode.vi"("TopLevelVI Path"=w5, "error in"=w1) -> ("error out"=→"error out":errorcluster)  [unwired: 9 in]
